vi "arrayI16.vi"(2 "Array In":i16[](array[numeric]), 3 "Base":i16) -> (0 "Array Out (not in place)":i16[](array[numeric]), 1 "Array Out":i16[](array[numeric]))   [LabVIEW 2012]
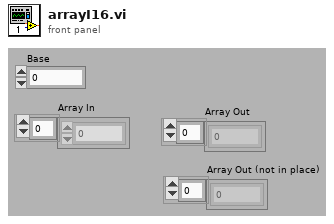
[diagram p1: front panel]
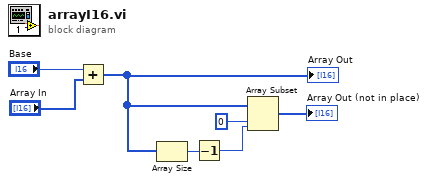
[diagram p0: block diagram]
diagram:
  n1 = Add(x="Base", y="Array In") -> (x+y=w1:i16[])
  "Array Out" <- w1
  n2 = Array Size(array=w1) -> (size(s)=w5:i32)
  n3 = Decrement(x=w5) -> (x-1=w6:i32)
  n4 = Array Subset(array=w1, index=0, length=w6) -> (→"Array Out (not in place)":i16[])
